vi "Get Port Status.vi"(8 "error in (no error)":errorcluster, 10 "Port":dbl, 11 "Cypress in":refnum<class "Cypress.lvclass">) -> (0 "error out":errorcluster, 3 "Cypress out":refnum<class "Cypress.lvclass">)   [LabVIEW 2020, in "Cypress.lvclass"]
uses:
  Cypress.lvclass
  c7faf52e-3808-4d03-9fab-3d2778e6b3bd.vi
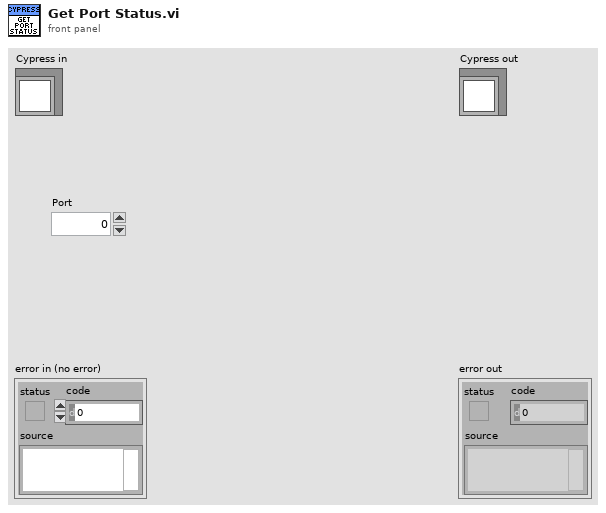
[diagram p1: front panel]
types:
  T1 = typedef "Serial device.lvclass/Brand combobox.ctl" = string
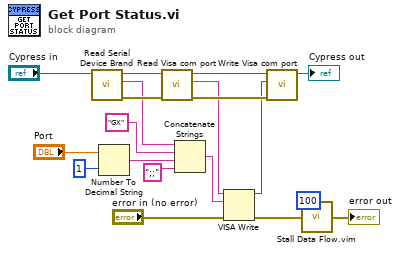
[diagram p0: block diagram]
diagram:
  n1 = call-dynamic "Read Serial Device Brand.vi"("Serial device in"="Cypress in") -> ("error out"=w11:errorcluster, "Serial Device Brand"=w8:T1, "Serial device out"=w12:refnum<class "Cypress.lvclass">)  [unwired: 8 in]
  n2 = Number To Decimal String(number="Port", width (-)=i16 1) -> (decimal integer string=w17:string)
  n3 = call-dynamic "Read Visa com port.vi"("error in (no error)"=w11, "Serial device in"=w12) -> ("error out"=w9:errorcluster, "Visa com port"=w7:string, "Serial device out"=w10:refnum<class "Cypress.lvclass">)  [unwired: 7 in]
  n4 = Concatenate Strings(w8, "GX" ("string"), w17, ";;" ("string")) -> (w18:string)
  n5 = VISA Write(VISA resource name=w7, write buffer=w18, error in (no error)="error in (no error)") -> (VISA resource name out=w6:refnum<visa-resource-name>, error out=w19:errorcluster)  [unwired: 1 out]
  n6 = call-dynamic "Write Visa com port.vi"("error in (no error)"=w9, "Visa com port"=w6, "Serial device in"=w10) -> ("Serial device out"=→"Cypress out":refnum<class "Cypress.lvclass">)  [unwired: 7 in, 1 out]
  n7 = call "Stall Data Flow.vim"("value in"=w19, "milliseconds to wait"=u32 100) -> ("value out"=→"error out":errorcluster)  [unwired: 1 out]
